vi "rad_Real-Time CPU Check.vi"(11 "Target settings in":T1 {"Primary NIC"."IP Address Request Mode" items=["Static"=1, "DHCP/Link-Local"=2, "Link-Local Only"=4, "DHCP Only"=8]}) -> (3 "Target settings out":T1 {"Primary NIC"."IP Address Request Mode" items=["Static"=1, "DHCP/Link-Local"=2, "Link-Local Only"=4, "DHCP Only"=8]})   [LabVIEW 2018]
uses:
  Targets/TypeDefs/rad_Target Information.ctl
  Targets/TypeDefs/rad_Target Network Settings.ctl
  <vilib>/nisyscfg/nisyscfg.lvlib
  <resource>/objmgr/motionsysapi.rc
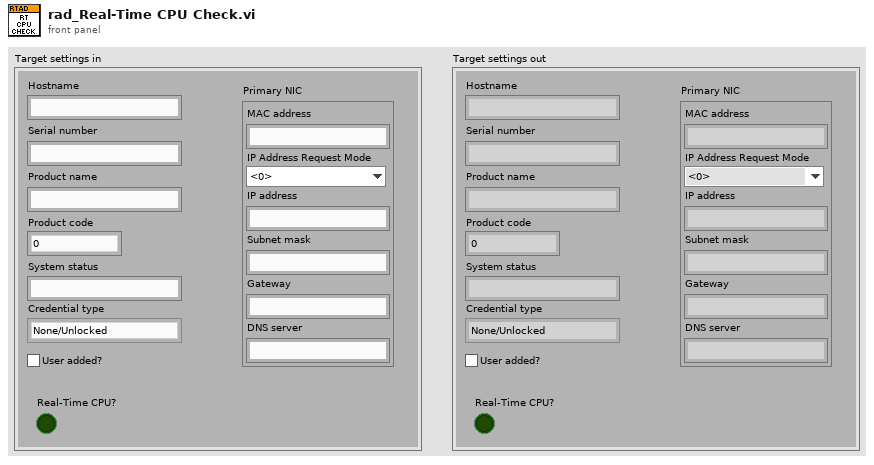
[diagram p1: front panel]
types:
  T1 = typedef "rad_Target Information.ctl" = cluster{"Hostname":string, "Serial number":string, "Product name":string, "Product code":i32, "System status":string, "Credential type":enum16{"None/Unlocked", "FTP Password", "NIAuth Credentials"}, "User added?":bool, "Primary NIC":T2, "Real-Time CPU?":bool}
  T2 = typedef "rad_Target Network Settings.ctl" = cluster{"MAC address":string, "IP Address Request Mode":i32, "IP address":string, "Subnet mask":string, "Gateway":string, "DNS server":string}
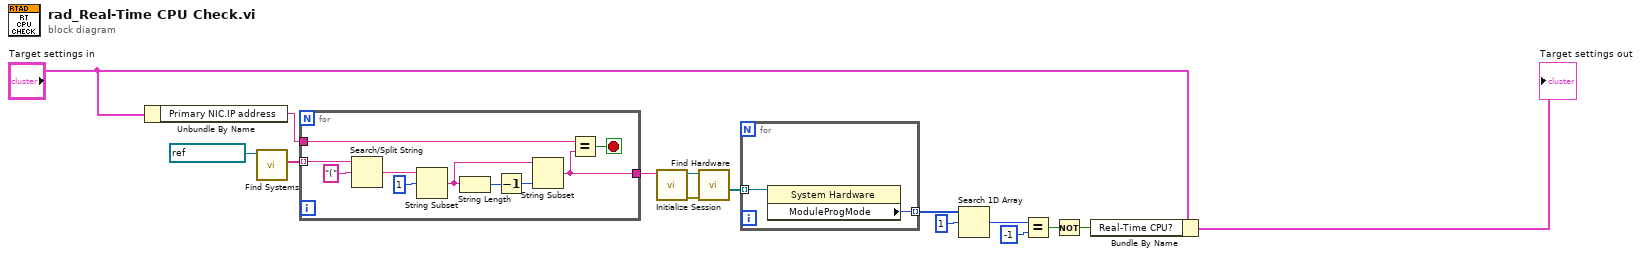
[diagram p0: block diagram]
diagram:
  n1 = Unbundle By Name("Target settings in") -> ("Primary NIC.IP address"=w5:string)
  n2 = call <vilib>:"Find Systems.vi"("Session in (localhost)"=refnum<k21> "localhost") -> ("Detected Systems"=w4:string[])  [unwired: 8 in, 2 out]
  n3 = for {
    tunnel: w4 -> [w25] mode=indexing
    tunnel: w5 -> [w18]
    tunnel: [w17] -> w6
    stop <- w16 stop-if-true
    n4 = Search/Split String(string=w25, search string/char (-)="(") -> (match + rest of string=w23:string)  [unwired: 1 in, 2 out]
    n5 = String Subset(string=w23, offset (0)=1) -> (substring=w21:string)  [unwired: 1 in]
    n6 = String Length(string=w21) -> (length=w20:i32)
    n7 = Decrement(x=w20) -> (x-1=w19:i32)
    n8 = String Subset(string=w21, length (rest)=w19) -> (substring=w17:string)  [unwired: 1 in]
    n9 = Equal?(x=w18, y=w17) -> (x = y?=w16:bool)
  }
  n10 = call <vilib>:"Initialize Session.vi"("Target (localhost)"=w6) -> ("error out"=w8:errorcluster, "Session out"=w7:refnum<k21>)  [unwired: 9 in]
  n11 = call <vilib>:"Find Hardware.vi"("error in (no error)"=w8, "Session in"=w7) -> ("Resources out"=w9:refnum<k20>[])  [unwired: 6 in, 3 out]
  n12 = for {
    tunnel: w9 -> [w27] mode=indexing
    tunnel: [w26] -> w10 mode=indexing
    n13 = property class="System Hardware"(reference=w27) -> ("ModuleProgMode"=w26:u32)  [unwired: 1 in, 2 out]
  }
  n14 = Search 1D Array(1D array=w10, element=u32 1) -> (index of element=w12:i32)  [unwired: 1 in]
  n15 = Equal?(x=w12, y=-1) -> (x = y?=w14:bool)
  n16 = Not(x=w14) -> (.not. x?=w15:bool)
  n17 = Bundle By Name(cluster="Target settings in", "Real-Time CPU?"=w15) -> (→"Target settings out":T1)
